vi "readThermoCouple.vi"() -> ()   [LabVIEW 2019]
panel:
  out "Numeric":dbl
  in  "stop":bool
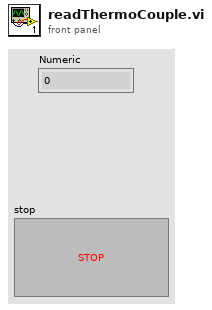
[diagram p1: front panel]
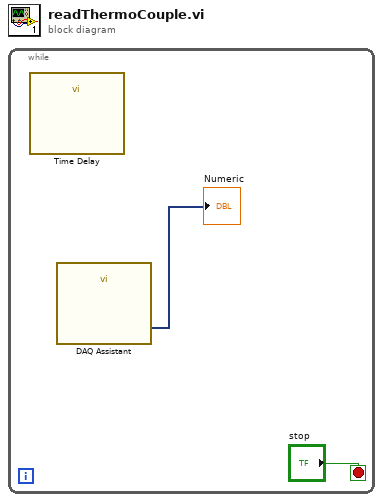
[diagram p0: block diagram]
diagram:
  n1 = while {
    stop <- "stop" stop-if-true
    n2 = call "Time Delay"() -> ()  [unwired: 11 in, 1 out]
    n3 = call "DAQ Assistant"() -> ("data"=→"Numeric":dynamicdata)  [unwired: 17 in, 2 out]
  }
